vi "CTR_to_DutyCycle.vi"(2 "LOW CTR":u32, 3 "HIGH CTR":u32) -> (0 "duty cycle fraction [0-1]":dbl, 1 "period [s]":dbl)   [LabVIEW 2013]
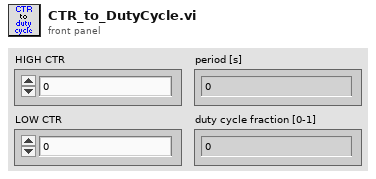
[diagram p1: front panel]
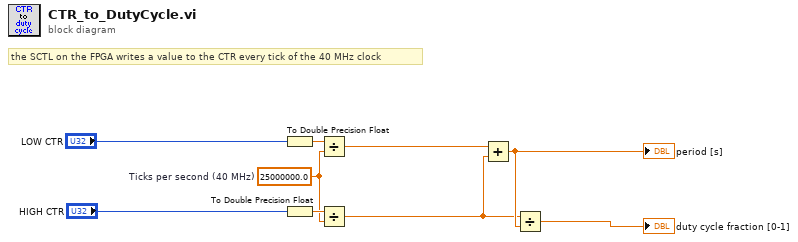
[diagram p0: block diagram]
diagram:
  w4 = 25000000.0  # Ticks per second (40 MHz)
  # "the SCTL on the FPGA writes a value to the CTR every tick of the 40 MHz clock"
  n1 = To Double Precision Float(number="LOW CTR") -> (double precision float=w5:dbl)
  n2 = To Double Precision Float(number="HIGH CTR") -> (double precision float=w6:dbl)
  n3 = Divide(x=w5, y=w4) -> (x/y=w3:dbl)
  n4 = Divide(x=w6, y=w4) -> (x/y=w2:dbl)
  n5 = Add(x=w3, y=w2) -> (x+y=w7:dbl)
  "period [s]" <- w7
  n6 = Divide(x=w2, y=w7) -> (x/y=→"duty cycle fraction [0-1]":dbl)
